vi "NEW_TOF_TO_NEW_LF.vi"(9 "NEXT TOF":bool[][](array[boolean]), 10 "Col":i32, 11 "Row":i32) -> (3 "Next LF":u32[][](array[numeric]))   [LabVIEW 2013]
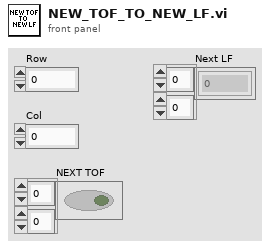
[diagram p1: front panel]
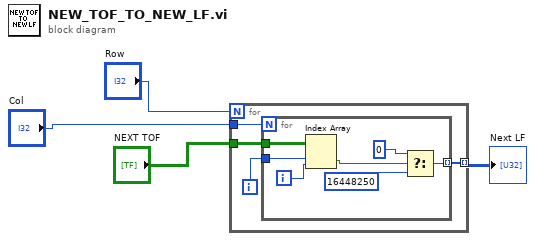
[diagram p0: block diagram]
diagram:
  n1 = for {
    N: "Row" -> [_]
    tunnel: "NEXT TOF" -> [w7]
    tunnel: [w6] -> w2 mode=indexing
    tunnel: "Col" -> [w5]
    i -> [w8]
    n2 = for {
      N: w5 -> [_]
      tunnel: w8 -> [w15]
      tunnel: w7 -> [w13]
      tunnel: [w12] -> w6 mode=indexing
      i -> [w14]
      n3 = Index Array(array=w13, index (row)=w15, index (col)=w14) -> (element=w11:bool)
      n4 = Select(t=u32 0 ("f"), s=w11, f=u32 16448250 ("y")) -> (s? t:f=w12:u32)
    }
  }
  "Next LF" <- w2
